vi "Calculate Frequency (Phase Correct Mode).vi"(9 "Clock Divisor":u32, 10 "TOP":dbl, 11 "Base Clock Frequency (Hz)":dbl) -> (3 "Frequency (Hz)":dbl)   [LabVIEW 2021]
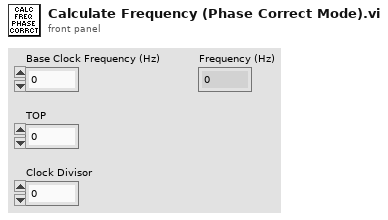
[diagram p1: front panel]
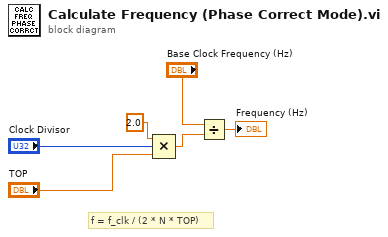
[diagram p0: block diagram]
diagram:
  # "f = f_clk / (2 * N * TOP)"
  n1 = Compound Arithmetic op=MULTIPLY(2.0 ("value"), "Clock Divisor", "TOP") -> (w2:dbl)
  n2 = Divide(x="Base Clock Frequency (Hz)", y=w2) -> (x/y=→"Frequency (Hz)":dbl)
